vi "Set NodeIDs.vi"(8 "error in (no error)":errorcluster, 10 "PLC Folder Names":string[](array[string]), 11 "OPC UA in":refnum<class "OPC UA.lvclass">) -> (0 "error out":errorcluster, 3 "OPC UA out":refnum<class "OPC UA.lvclass">)   [LabVIEW 2019, in "OPC UA.lvlib" / "OPC UA.lvclass"]
uses:
  OPC UA.lvclass
  OPC UA.lvclass/OPC UA.ctl
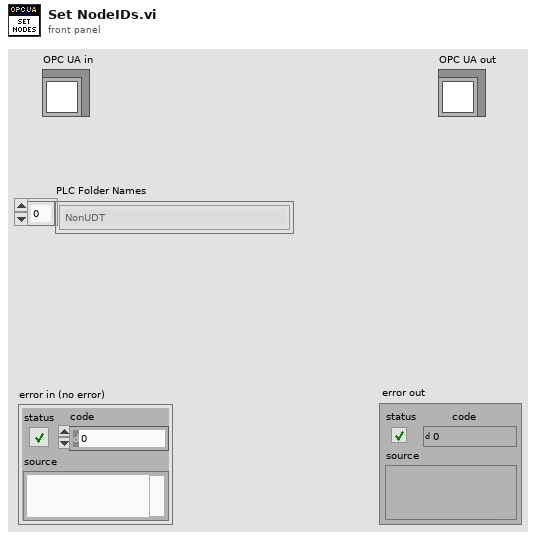
[diagram p1: front panel]
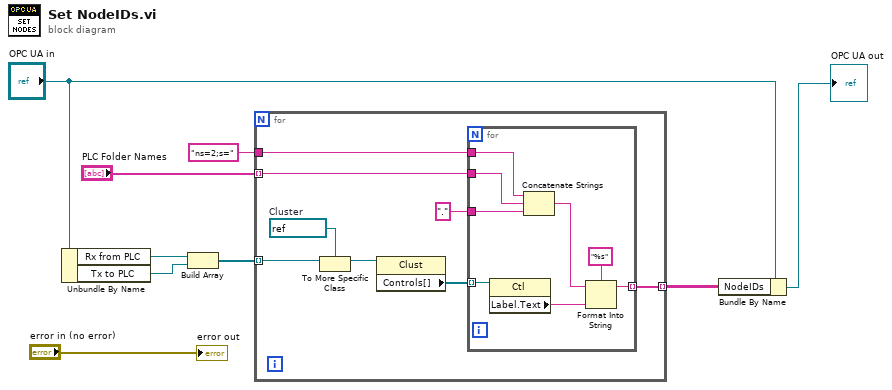
[diagram p0: block diagram]
diagram:
  n1 = Unbundle By Name("OPC UA in") -> ("Rx from PLC"=w3:refnum<vi>, "Tx to PLC"=w2:refnum<vi>)
  n2 = Build Array(w3, w2) -> (w1:refnum<vi>[])
  n3 = for {
    tunnel: "ns=2;s=" ("format string") -> [w17]
    tunnel: [w16] -> w7 mode=indexing
    tunnel: "PLC Folder Names" -> [w15] mode=indexing
    tunnel: w1 -> [w11] mode=indexing
    w13 = refnum<vi> refnum  # Cluster
    n4 = To More Specific Class(target class=w13, reference=w11) -> (specific class reference=w12:refnum<vi>)  [unwired: 1 in, 1 out]
    n5 = property class="Clust"(reference=w12) -> ("Controls[]"=w14:refnum<vi>[])  [unwired: 1 in, 2 out]
    n6 = for {
      tunnel: w14 -> [w25] mode=indexing
      tunnel: w15 -> [w21]
      tunnel: [w22] -> w16 mode=indexing
      tunnel: w17 -> [w20]
      tunnel: "." ("Deliminated Char") -> [w18]
      n7 = property class="Ctl"(reference=w25) -> ("Label.Text"=w24:string)  [unwired: 1 in, 2 out]
      n8 = Concatenate Strings(w20, w21, w18) -> (w19:string)
      n9 = Format Into String(format string="%s", initial string=w19, w24) -> (resulting string=w22:string)  [unwired: 1 in, 1 out]
    }
  }
  n10 = Bundle By Name(cluster="OPC UA in", "NodeIDs"=w7) -> (→"OPC UA out":refnum<class "OPC UA.lvclass">)
  "error out" <- "error in (no error)"
